vi "DotNETCam_Start.vi"(8 "ErrorIn":errorcluster, 10 "CmdData":variant, 11 "DotNETCamIn":refnum<class>) -> (0 "ErrorOut":errorcluster, 2 "ReplyData":variant, 3 "DotNETCamOut":refnum<class>, 4 "Exit":bool)   [LabVIEW 2021, in "DotNETCam.lvclass"]
uses:
  DotNETCam.lvclass
  DotNETCam.lvclass/DotNETCam.ctl
  State.ctl
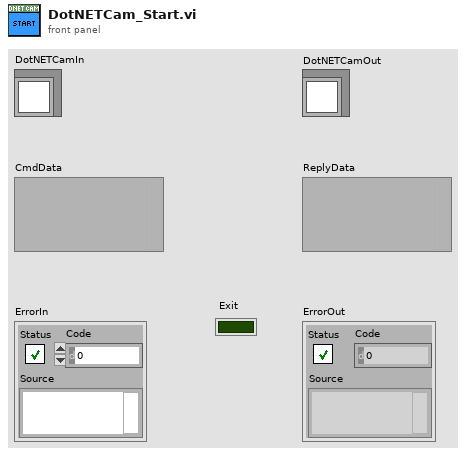
[diagram p1: front panel]
types:
  T1 = enum32{"Invalid", "Standard", "Closed", "Hidden", "Minimized", "Maximized"}
  T2 = typedef "DotNETCam.lvclass/State.ctl" = enum16{"Idle", "Acquiring"}
  T3 = cluster{"posX":i32, "posY":i32, "nWidth":i32, "nHeight":i32}
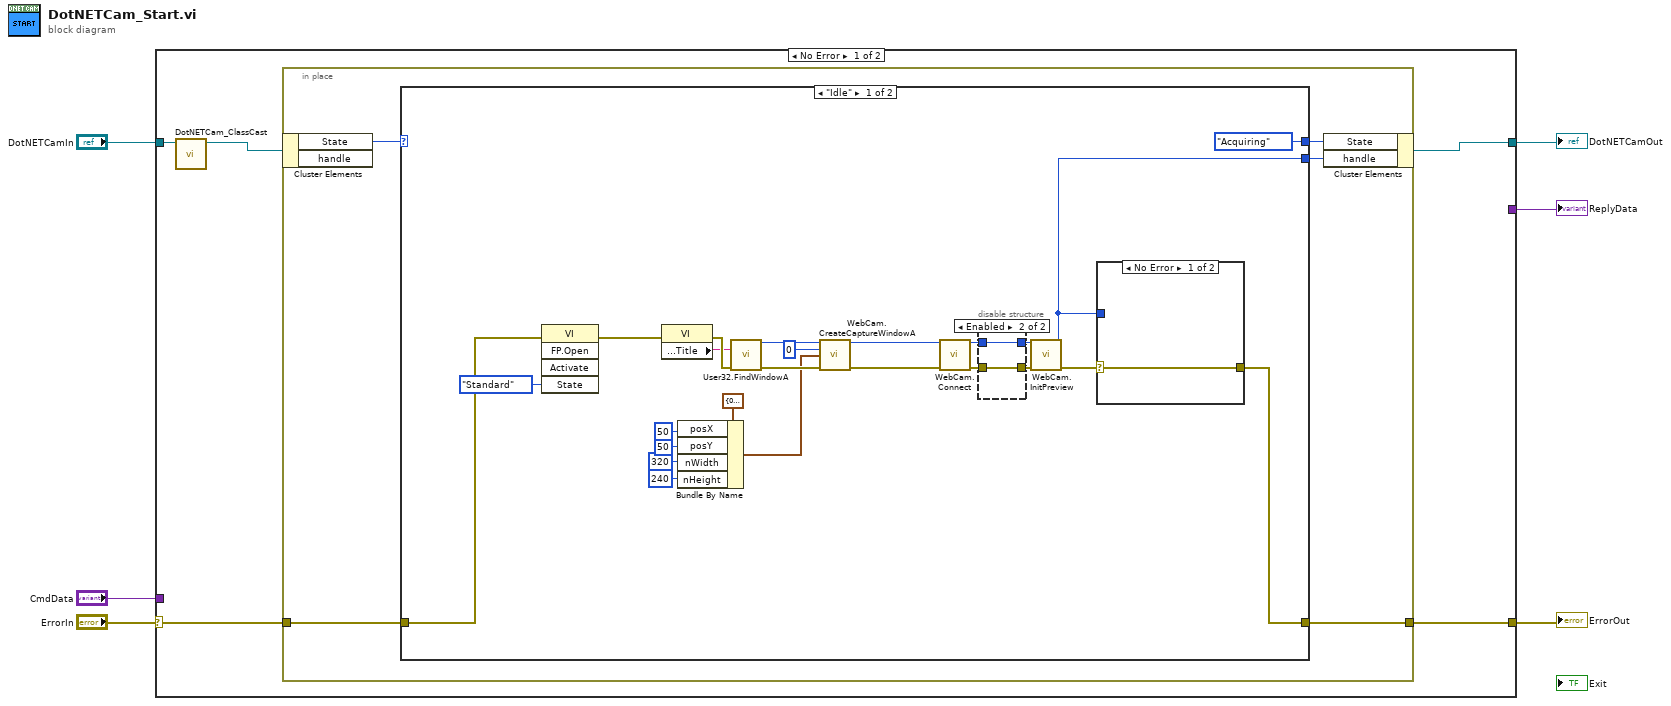
[diagram p0: block diagram]
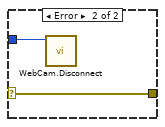
[diagram p2: hidden frame]
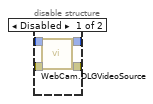
[diagram p3: hidden frame]
diagram:
  n1 = case shown="No Error" "ErrorIn" {
    selector: "ErrorIn" -> [w11 w54]
    tunnel: [w10 w54] -> w5
    tunnel: [_ w53] -> w3
    tunnel: "CmdData" -> [_ w53]
    tunnel: "DotNETCamIn" -> [w9 w52]
    tunnel: [w7 w52] -> w1
    frame No Error {
      n2 = call "DotNETCam_ClassCast.vi"("DotNETCamIn"=w9) -> ("DotNETCamOut"=w8:refnum<class "DotNETCam.lvclass">)  [unwired: 10 in]
      n3 = in-place {
        in-place-border: w11 -> [w16]
        in-place-border: [w15] -> w10
        n4 = in-place-cluster #1(w8) -> ("State"=w14:T2)  [unwired: 1 out]
        n5 = case shown="\"Idle\"" w14 {
          selector: w14 -> [_ w50]
          tunnel: [w33 w51] -> w15
          tunnel: w16 -> [w35 w51]
          tunnel: [State."Acquiring" ("State") w50] -> w13
          tunnel: [w18 _] -> w12
          frame "Idle" {
            n6 = invoke class="VI" method="FP.Open"(error in=w35, "State"=T1."Standard") -> (error out=w32:errorcluster)  [unwired: 3 in, 4 out]
            n7 = property class="VI"(error in=w32) -> (error out=w37:errorcluster, "Front Panel Window:Title"=w21:string)  [unwired: 1 in, 1 out]
            n8 = Bundle By Name(cluster=T3 {"posX"=0, "posY"=0, "nWidth"=0, "nHeight"=0} ("rect"), "posX"=50 ("nWidth"), "posY"=50 ("nWidth"), "nWidth"=320, "nHeight"=240 ("nWidth")) -> (w22:T3)
            n9 = call "User32.FindWindowA.vi"("LpWindowName"=w21, "ErrorIn"=w37) -> ("Hwnd"=w24:i32, "ErrorOut"=w38:errorcluster)  [unwired: 12 in]
            n10 = call "WebCam.CreateCaptureWindowA.vi"("Handle"=w24, "NID"=0 ("nID"), "Rect"=w22, "ErrorIn"=w38) -> ("HandleOut"=w20:i32, "ErrorOut"=w36:errorcluster)  [unwired: 10 in]
            n11 = call "WebCam.Connect.vi"("Handle"=w20, "ErrorIn"=w36) -> ("HandleOut"=w31:i32, "ErrorOut"=w40:errorcluster)  [unwired: 12 in]
            n12 = disable-structure shown="Enabled" {
              disable-tunnel: w31 -> [w45 w48]
              disable-tunnel: w40 -> [w47 w49]
              disable-tunnel: [w46 w49] -> w39
              disable-tunnel: [w44 w48] -> w30
              frame Disabled {
                n13 = call "WebCam.DLGVideoSource.vi"("Handle"=w45, "ErrorIn"=w47) -> ("HandleOut"=w44:i32, "ErrorOut"=w46:errorcluster)  [unwired: 12 in]
              }
              frame Enabled {
              }
            }
            n14 = call "WebCam.InitPreview.vi"("Handle"=w30, "ErrorIn"=w39) -> ("HandleOut"=w18:i32, "ErrorOut"=w34:errorcluster)  [unwired: 12 in]
            n15 = case shown="No Error" w34 {
              selector: w34 -> [w41 w43]
              tunnel: w18 -> [_ w42]
              tunnel: [w41 w43] -> w33
              frame No Error {
              }
              frame Error {
                n16 = call "WebCam.Disconnect.vi"("Handle"=w42) -> ()  [unwired: 14 in, 1 out]
              }
            }
          }
          frame "Acquiring" {
          }
        }
        n17 = in-place-cluster #1("State"=w13, "handle"=w12) -> (w7:refnum<class "DotNETCam.lvclass">)
      }
    }
    frame Error {
    }
  }
  "ErrorOut" <- w5
  "DotNETCamOut" <- w1
  "ReplyData" <- w3
